vi "Simple TCP - Server.vi"() -> ()   [LabVIEW 2015]
doc: "Demonstrates how to set up a basic TCP connection, send data to the specified port once a connection has been established, and terminate the connection once the data has been sent. This VI is designed to stop if the TCP connection is terminated. The data sent in this example is an array of random numbers."
uses:
  <vilib>/sound2/lvsound2.llb/Sampling Mode.ctl
  <vilib>/sound2/lvsound2.llb/Sound Data Format.ctl
  <vilib>/sound2/lvsound2.llb/Sound Input Read (DBL).vi
panel:
  in  "Device ID":u32 format="%.0x"
  in  "Number of Samples/ch":i32=5000
  in  "Client Closed":string="The client VI closed the connection."
  out "Waveform Graph":dbl[](graph)
  in  "Stop":bool
  # "Overview: Demonstrates the use of the TCP functions to initialize a TCP server that can send data to a client VI.\nInstructions:\n1. Run the VI.\n2. Open Simple TCP - Client.vi and follow the instructions on its front panel. Note that if you wait longer than 30 seconds to do this after running this VI, it will time out.\n3. Click Stop to stop the VI. Note that if you stop the client VI, this VI will stop automatically."
  # "Microphone:"
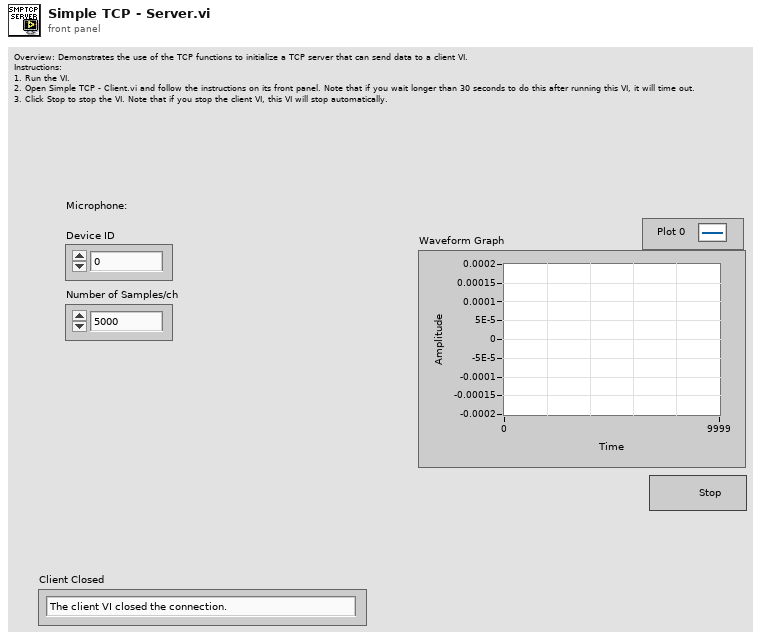
[diagram p1: front panel]
types:
  T1 = typedef "Sound Data Format.ctl" = cluster{"sample rate (S/s)":dbl, "number of channels":i32, "bits per sample":i32}
  T2 = typedef "Sampling Mode.ctl" = i32
  T3 = typedef "Sound Input Task ID.ctl" = u32
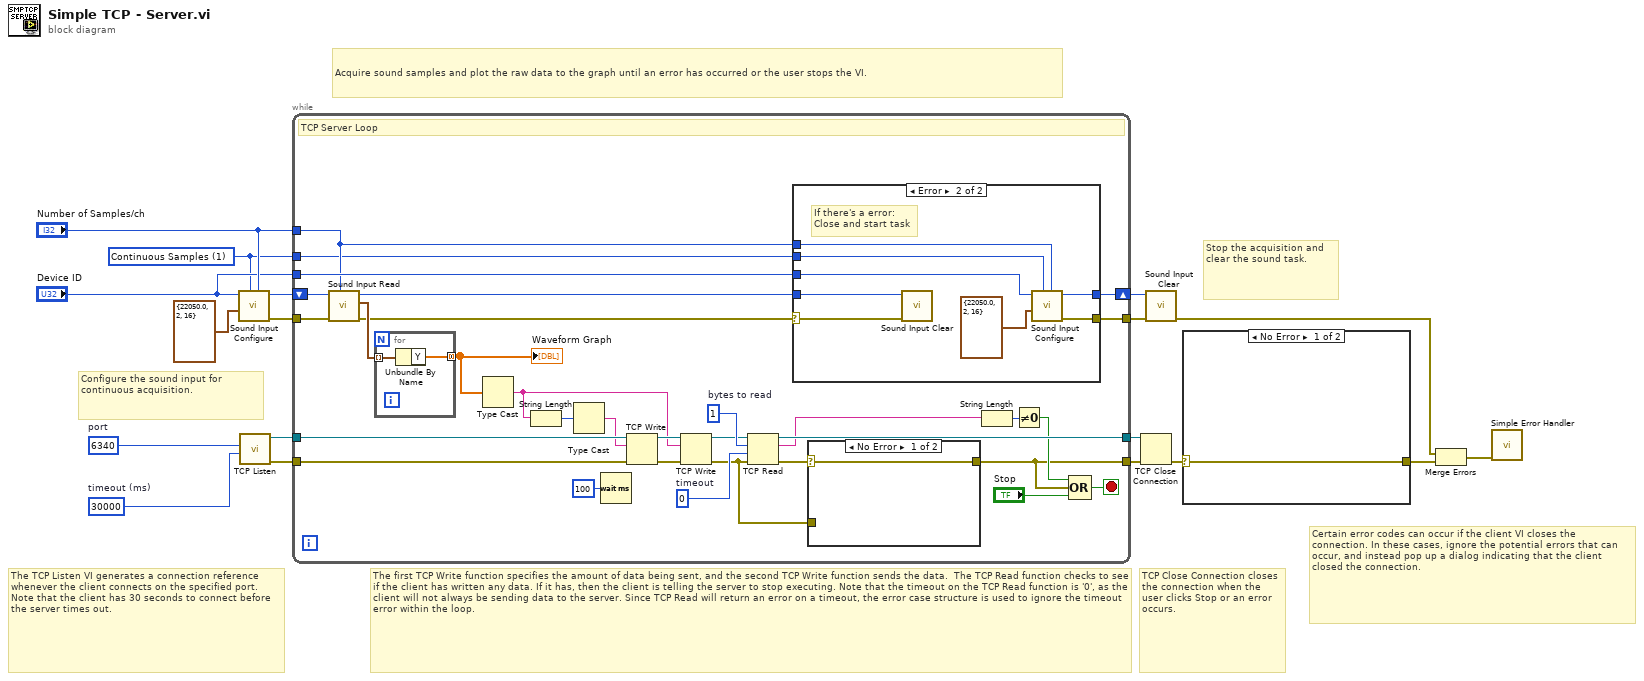
[diagram p0: block diagram]
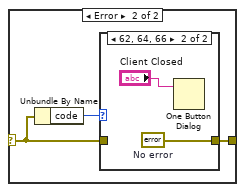
[diagram p2: hidden frame]
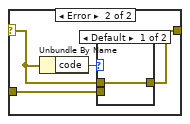
[diagram p5: hidden frame]
diagram:
  w1 = T2 1 items=["Finite Samples", "Continuous Samples"] ("sample mode")
  w11 = u16 6340  # port
  w12 = 30000  # timeout (ms)
  # "Acquire sound samples and plot the raw data to the graph until an error has occurred or the user stops the VI."
  # "Stop the acquisition and clear the sound task."
  # "Configure the sound input for continuous acquisition."
  # "TCP Close Connection closes the connection when the user clicks Stop or an error occurs."
  # "The TCP Listen VI generates a connection reference whenever the client connects on the specified port. Note that the client has 30 seconds to connect before the server times out."
  # "Certain error codes can occur if the client VI closes the connection. In these cases, ignore the potential errors that can occur, and instead pop up a dialog indicating that the client closed the connection."
  # "The first TCP Write function specifies the amount of data being sent, and the second TCP Write function sends the data.  The TCP Read function checks to see if the client has written any data. If it has, then the client is telling the server to stop executing. Note that the timeout on the TCP Read function is '0', as the client will not always be sending data to the server. Since TCP Read will return an error on a timeout, the error case structure is used to ignore the timeout error within the loop."
  n1 = call <vilib>:"Sound Input Configure.vi"("number of samples/ch"="Number of Samples/ch", "sample mode"=w1, "sound format"=T1 {"sample rate (S/s)"=22050.0, "number of channels"=2, "bits per sample"=16} ("Sound Format"), "device ID"="Device ID") -> ("error out"=w8:errorcluster, "task ID"=w9:T3)  [unwired: 6 in]
  n2 = call <vilib>:"TCP Listen.vi"("timeout ms (wait forever: -1)"=w12, "port"=w11) -> ("error out"=w13:errorcluster, "connection ID"=w14:refnum<k5>)  [unwired: 5 in, 3 out]
  n3 = while {
    tunnel: [w31] -> w17
    tunnel: [w37] -> w18
    tunnel: w14 -> [w49]
    tunnel: w13 -> [w41]
    tunnel: w8 -> [w28]
    tunnel: "Number of Samples/ch" -> [w20]
    shift-right: [w23] -> w3
    shift-left: w9 -> [w29]
    tunnel: [w22] -> w4
    tunnel: "Device ID" -> [w21]
    tunnel: w1 -> [w19]
    stop <- w42 stop-if-true
    w36 = 0  # timeout
    w39 = 1  # bytes to read
    # "TCP Server Loop"
    n4 = call-poly <vilib>:"Sound Input Read.vi"("number of samples/ch"=w20, "error in (no error)"=w28, "task ID"=w29) -> ("error out"=w25:errorcluster, "data"=w27:waveform(dbl)[], "task ID out"=w24:T3)  [unwired: 6 in]
    n5 = for {
      tunnel: w27 -> [w61] mode=indexing
      tunnel: [w60] -> w26 mode=concatenating
      n6 = Unbundle By Name(w61) -> ("Y"=w60:dbl[])
    }
    "Waveform Graph" <- w26
    n7 = Type Cast(x=w26) -> (*(type *) &x=w44:string)  [unwired: 1 out]
    n8 = String Length(string=w44) -> (length=w46:i32)
    n9 = Type Cast(x=w46) -> (*(type *) &x=w45:string)  [unwired: 1 out]
    n10 = Wait (ms)(milliseconds to wait=u32 100) -> ()  [unwired: 1 out]
    n11 = TCP Write(connection ID=w49, data in=w45, error in (no error)=w41) -> (connection ID out=w48:refnum<k5>, error out=w47:errorcluster)  [unwired: 2 out]
    n12 = TCP Write(connection ID=w48, data in=w44, error in (no error)=w47) -> (connection ID out=w38:refnum<k5>, error out=w30:errorcluster)  [unwired: 2 out]
    n13 = TCP Read(connection ID=w38, bytes to read=w39, error in (no error)=w30, 9:w36) -> (connection ID out=w37:refnum<k5>, data out=w34:string, error out=w32:errorcluster)  [unwired: 1 out]
    n14 = case shown="Error" w25 {
      selector: w25 -> [w50 w59]
      tunnel: w24 -> [w51 w58]
      tunnel: [w51 w57] -> w23
      tunnel: [w50 w56] -> w22
      tunnel: w21 -> [_ w55]
      tunnel: w20 -> [_ w54]
      tunnel: w19 -> [_ w53]
      frame No Error {
      }
      frame Error {
        # "If there's a error:\nClose and start task"
        n15 = call <vilib>:"Sound Input Clear.vi"("error in (no error)"=w59, "task ID"=w58) -> ()  [unwired: 9 in, 1 out]
        n16 = call <vilib>:"Sound Input Configure.vi"("number of samples/ch"=w54, "sample mode"=w53, "sound format"=T1 {"sample rate (S/s)"=22050.0, "number of channels"=2, "bits per sample"=16} ("Sound Format"), "device ID"=w55) -> ("error out"=w56:errorcluster, "task ID"=w57:T3)  [unwired: 6 in]
      }
    }
    n17 = case shown="No Error" w32 {
      selector: w32 -> [w62 w65]
      tunnel: [w62 w63] -> w31
      tunnel: w30 -> [_ w64]
      frame No Error {
      }
      frame Error {
        n18 = Unbundle By Name(w65) -> ("code"=w66:i32)
        n19 = case shown="Default" w66 {
          tunnel: w65 -> [w67 _]
          tunnel: w64 -> [_ w68]
          tunnel: [w67 w68] -> w63
          frame Default {
          }
          frame 56 {
          }
        }
      }
    }
    n20 = String Length(string=w34) -> (length=w35:i32)
    n21 = Not Equal To 0?(x=w35) -> (x != 0?=w33:bool)
    n22 = Compound Arithmetic op=OR(w33, w31, "Stop") -> (w42:bool)
  }
  n23 = TCP Close Connection(connection ID=w18, error in (no error)=w17) -> (error out=w16:errorcluster)  [unwired: 2 out]
  n24 = call <vilib>:"Sound Input Clear.vi"("error in (no error)"=w4, "task ID"=w3) -> ("error out"=w6:errorcluster)  [unwired: 9 in]
  n25 = case shown="No Error" w16 {
    selector: w16 -> [w69 w71]
    tunnel: [w69 w70] -> w15
    frame No Error {
    }
    frame Error {
      n26 = Unbundle By Name(w71) -> ("code"=w72:i32)
      n27 = case shown="62, 64, 66" w72 {
        tunnel: w71 -> [w73 _]
        tunnel: [w73 w75] -> w70
        frame Default {
        }
        frame 62, 64, 66 {
          w75 = errorcluster {"status"=FALSE, "code"=0, "source"=""}  # No error
          n28 = One Button Dialog(message="Client Closed") -> ()  [unwired: 1 in, 1 out]
        }
      }
    }
  }
  n29 = Merge Errors(w6, w15) -> (w7:errorcluster)
  n30 = call <vilib>:"Simple Error Handler.vi"("error in (no error)"=w7) -> ()  [unwired: 1 in, 8 out]
